vi "Format Error Terminals.vi"(8 "error in (no error)":errorcluster, 11 "VI Ref":refnum<vi>) -> (0 "error out":errorcluster, 2 "Save?":bool, 3 "VI Ref out":refnum<vi>)   [LabVIEW 2020, in "Code Cleanup.lvlib"]
uses:
  Code Cleanup.lvlib
  <vilib>/Utility/traverseref.llb/VI Scripting - Traverse.lvlib
  <vilib>/Utility/traverseref.llb/TRef TravTarget.ctl
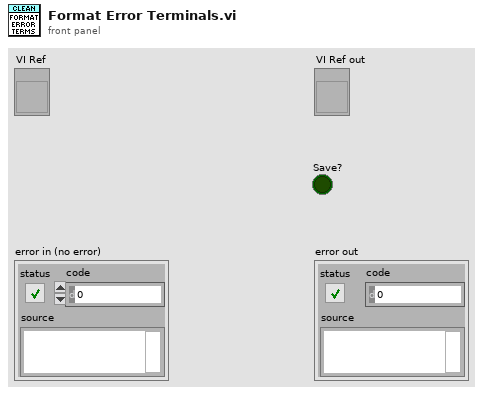
[diagram p1: front panel]
types:
  T1 = typedef "TRef TravTarget.ctl" = enum16{"FP", "BD", "Other"}
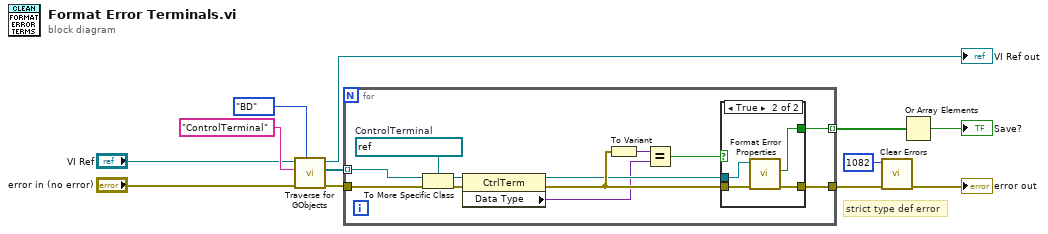
[diagram p0: block diagram]
diagram:
  # "strict type def error"
  n1 = call <vilib>:"Traverse for GObjects.vi"("Traverse Target"=TRef_TravTarget."BD", "error in (no error)"="error in (no error)", "Class Name"="ControlTerminal", "VI Refnum"="VI Ref") -> ("error out"=w9:errorcluster, "References"=w8:refnum<vi>[], "dup VI Refnum"=→"VI Ref out":refnum<vi>)  [unwired: 4 in, 1 out]
  n2 = for {
    tunnel: w8 -> [w24] mode=indexing
    tunnel: [w13] -> w4 mode=indexing
    tunnel: w9 -> [w20]
    tunnel: [w16] -> w6
    w23 = refnum<vi> refnum  # ControlTerminal
    n3 = To More Specific Class(target class=w23, reference=w24, error in=w20) -> (specific class reference=w22:refnum<vi>, error out=w21:errorcluster)
    n4 = property class="CtrlTerm"(reference=w22, error in=w21) -> (reference out=w15:refnum<vi>, error out=w18:errorcluster, "Data Type"=w14:variant)
    n5 = To Variant(anything=w18) -> (Variant=w19:variant)
    n6 = Equal?(x=w19, y=w14) -> (x = y?=w17:bool)
    n7 = case shown="True" w17 {
      tunnel: w18 -> [w25 w29]
      tunnel: [w25 w28] -> w16
      tunnel: w15 -> [_ w27]
      tunnel: [_ w26] -> w13
      frame False {
      }
      frame True {
        n8 = call "Format Error Properties.vi"("error in (no error)"=w29, "CtrlTerm Ref"=w27) -> ("error out"=w28:errorcluster, "Changed?"=w26:bool)  [unwired: 8 in]
      }
    }
  }
  n9 = call <vilib>:"Clear Errors.vi"("error in (no error)"=w6, "specific error code to clear (0: all)"=1082) -> ("error out"=→"error out":errorcluster)  [unwired: 4 in, 1 out]
  n10 = Or Array Elements(Boolean array=w4) -> (logical OR=→"Save?":bool)
